vi "PIDAutoTune_SetTuningArguments.vi"(4 "Long Ave Time":i32=6, 5 "Controller Constant Type":T1(ring)=enum."Ziegler Nicols - Slow", 6 "Newest Avg Time":i32=1, 7 "Type of Controller":enum16{"P", "PI", "PID"}(ring)=enum."PI", 8 "Plant Tolerance":dbl=0.001, 9 "Tuning Tolerance":dbl=0.001, 10 "Kn":dbl=1.0, 11 "CO Offset":dbl=0.25) -> (3 "Configuration Parameters":T2={"Controller Constant Type"=enum."Ziegler Nicols - Normal", "Type of Controller"=enum."PI", "CO Offset"=0.25, "Kn"=1.0, "Tuning Tolerance"=0.001, "Plant Tolerance"=0.001, "Newest Avg Time "=1, "Long Ave Time"=6})   [LabVIEW 2019, in "Trajectory_Library.lvlib"]
uses:
  Trajectory_Library.lvlib
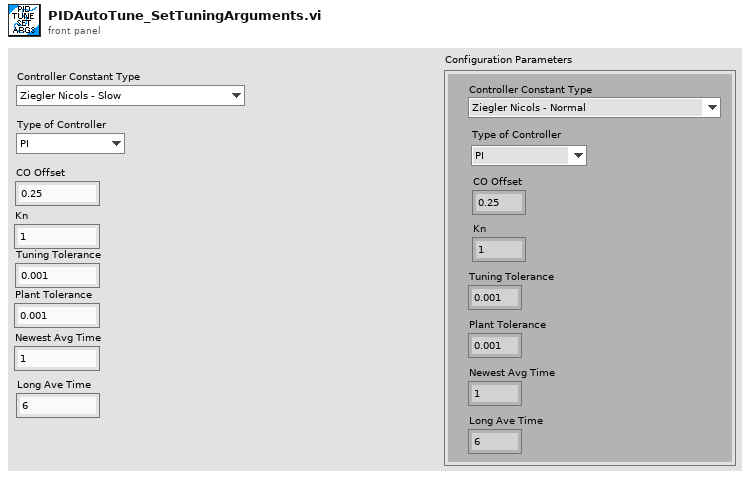
[diagram p1: front panel]
types:
  T1 = enum16{"Ziegler Nicols - Fast", "Ziegler Nicols - Normal", "Ziegler Nicols - Slow", "CHR regulator - 0% overshoot", "CHR regulator - 20% overshoot", "CHR servo - 0 % overshoot", "CHR servo - 20% overshoot"}
  T2 = cluster{"Controller Constant Type":enum16{"Ziegler Nicols - Fast", "Ziegler Nicols - Normal", "Ziegler Nicols - Slow", "CHR regulator - 0% overshoot", "CHR regulator - 20% overshoot", "CHR servo - 0 % overshoot", "CHR servo - 20% overshoot"}, "Type of Controller":enum16{"P", "PI", "PID"}, "CO Offset":dbl, "Kn":dbl, "Tuning Tolerance":dbl, "Plant Tolerance":dbl, "Newest Avg Time ":i32, "Long Ave Time":i32}
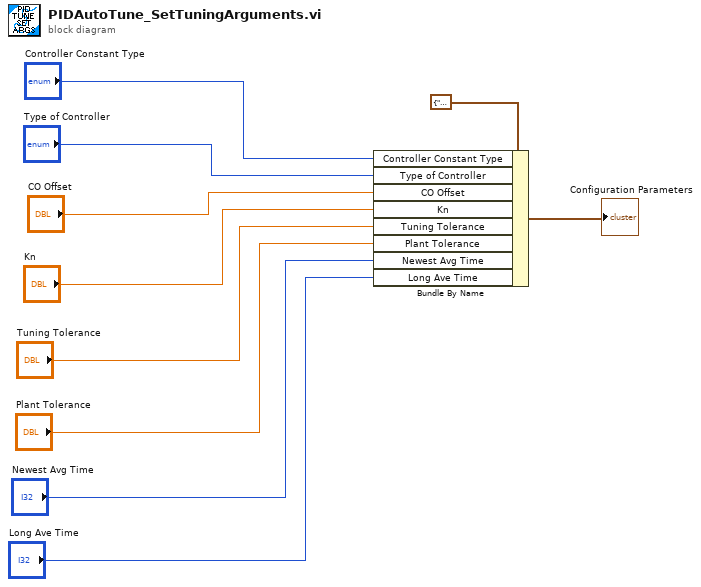
[diagram p0: block diagram]
diagram:
  n1 = Bundle By Name(cluster=T2 {"Controller Constant Type"=enum."Ziegler Nicols - Normal", "Type of Controller"=enum."PI", "CO Offset"=0.25, "Kn"=1.0, "Tuning Tolerance"=0.001, "Plant Tolerance"=0.001, "Newest Avg Time "=1, "Long Ave Time"=6} ("Tuning Parameters 2"), "Controller Constant Type"="Controller Constant Type", "Type of Controller"="Type of Controller", "CO Offset"="CO Offset", "Kn"="Kn", "Tuning Tolerance"="Tuning Tolerance", "Plant Tolerance"="Plant Tolerance", "Newest Avg Time"="Newest Avg Time", "Long Ave Time"="Long Ave Time") -> (→"Configuration Parameters":T2)
